vi "RecipeFile_Maker.vi"() -> ()   [LabVIEW 2014]
uses:
  <vilib>/Utility/file.llb/Write To Spreadsheet File (string).vi
panel:
  in  "RFSA_SettingFile_Path":path=path "C:/Gyuwon_Folder/SourceCodeFolder/1005_Gyu_RF_SourceProject_Msg/___SystemFiles/RFSA_Default_Setting.csv"
  in  "RFSG_SettingFile_Path":path=path "C:/Gyuwon_Folder/SourceCodeFolder/1005_Gyu_RF_SourceProject_Msg/___SystemFiles/RFSG_Default_Setting.csv"
  in  "RFSA_State":u16(ring) items=["RFSA_Init", "RFSA_Init_Servo", "Config_RFSA_AcqType_Vertical", "Config_RFSA_IQ_Acq", "Config_RFSA_Spectrum_Acq", "Config_RFSA_Trigger", "RFSA_Initiate", "RFSA_Fetch_IQ", "RFSA_Acq_Read_Spectrum", "RFSA_Acq_Read_IQ", "RFSA_Stop", "RFSA_Close", "Wait_Cmd", "Send_Cmd", "Exit"]
  in  "RFSG_State":u16(ring) items=["RFSG_Init", "RFSG_Init_Servo", "Config_ScriptWfm", "Config_Freq_Power_ExtGain", "Config_RFSG_Mode_CW", "Config_RFSG_Mode_Script", "RFSG_Write_Script", "RFSG_Initiate", "RFSG_Stop", "RFSG_Close", "Wait_Cmd", "Send_Cmd", "Exit"]
  in  "RFSA_Data":u16[](array[ring])=[0, 3, 1, 0, 0, 0] items=["None", "Config_RFSA_IQ_Acq", "Config_RFSA_Spectrum_Acq", "Config_RFSA_Vertical", "Config_RFSG"]
  in  "RFSA":u16[](array[ring])=[0, 2, 3, 5, 6, 7] items=["RFSA_Init", "RFSA_Init_Servo", "Config_RFSA_AcqType_Vertical", "Config_RFSA_IQ_Acq", "Config_RFSA_Spectrum_Acq", "Config_RFSA_Trigger", "RFSA_Initiate", "RFSA_Fetch_IQ", "RFSA_Acq_Read_Spectrum", "RFSA_Acq_Read_IQ", "RFSA_Stop", "RFSA_Close", "Wait_Cmd", "Send_Cmd", "Exit"]
  in  "RFSG_Data":u16[](array[ring])=[0, 4, 0, 0, 4, 0] items=["None", "Config_RFSA_IQ_Acq", "Config_RFSA_Spectrum_Acq", "Config_RFSA_Vertical", "Config_RFSG"]
  in  "RFSG":u16[](array[ring])=[0, 3, 2, 5, 6, 7] items=["RFSG_Init", "RFSG_Init_Servo", "Config_ScriptWfm", "Config_Freq_Power_ExtGain", "Config_RFSG_Mode_CW", "Config_RFSG_Mode_Script", "RFSG_Write_Script", "RFSG_Initiate", "RFSG_Stop", "RFSG_Close", "Wait_Cmd", "Send_Cmd", "Exit"]
  # "[ State 목록을 차후 변경될 때를 대비하여 enum으로 할 필요 있음 ]"
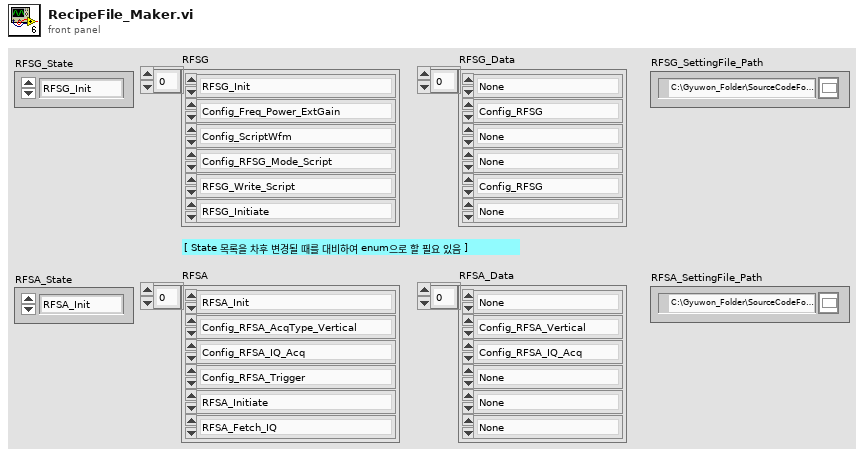
[diagram p1: front panel]
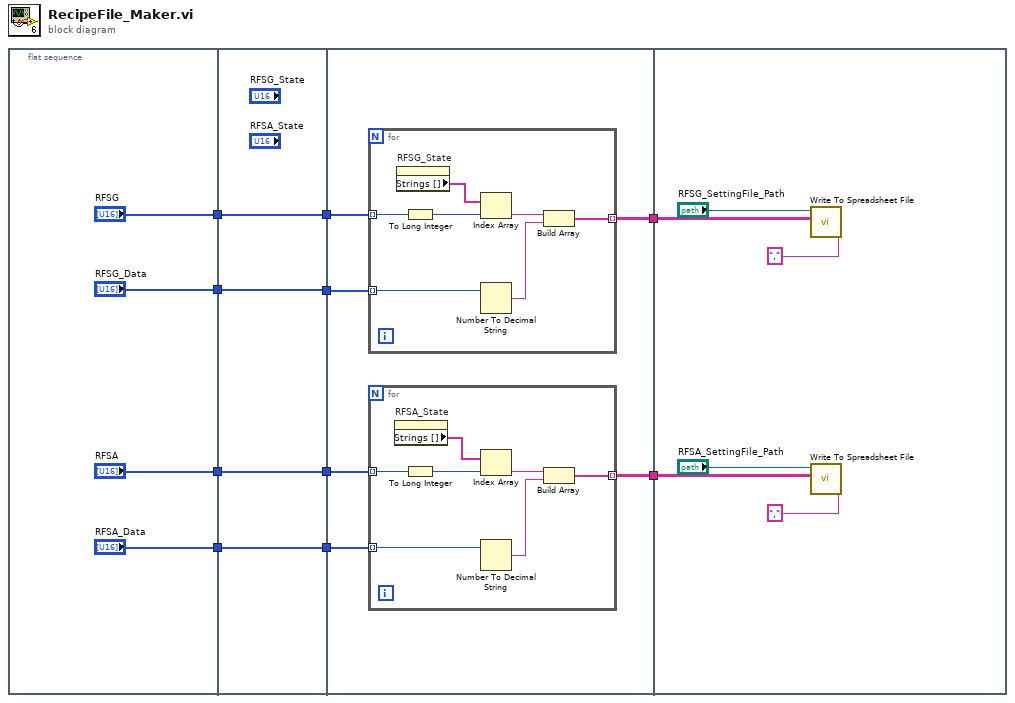
[diagram p0: block diagram]
diagram:
  n1 = flat-sequence {
    tunnel: ["RFSG"] -> w10
    tunnel: ["RFSG_Data"] -> w8
    tunnel: ["RFSA"] -> w5
    tunnel: ["RFSA_Data"] -> w1
    tunnel: w10 -> [w18]
    tunnel: [w18] -> w9
    tunnel: w8 -> [w17]
    tunnel: [w17] -> w7
    tunnel: w5 -> [w16]
    tunnel: [w16] -> w4
    tunnel: [w15] -> w2
    tunnel: w1 -> [w15]
    tunnel: w9 -> [w24]
    tunnel: w7 -> [w23]
    tunnel: [w22] -> w6
    tunnel: w4 -> [w21]
    tunnel: [w20] -> w3
    tunnel: w2 -> [w19]
    tunnel: w6 -> [w44]
    tunnel: w3 -> [w40]
    frame #0 {
    }
    frame #1 {
    }
    frame #2 {
      n2 = for {
        tunnel: w24 -> [w37] mode=indexing
        tunnel: w23 -> [w35] mode=indexing
        tunnel: [w32] -> w22 mode=indexing
        n3 = property on="RFSG_State" class="Ring (strict)"() -> ("Strings []"=w38:string[])  [unwired: 2 in, 2 out]
        n4 = To Long Integer(number=w37) -> (32bit integer=w36:i32)
        n5 = Index Array(array=w38, index=w36) -> (element=w34:string)
        n6 = Number To Decimal String(number=w35) -> (decimal integer string=w33:string)  [unwired: 1 in]
        n7 = Build Array(w34, w33) -> (w32:string[])
      }
      n8 = for {
        tunnel: w21 -> [w31] mode=indexing
        tunnel: w19 -> [w29] mode=indexing
        tunnel: [w26] -> w20 mode=indexing
        n9 = property on="RFSA_State" class="Ring (strict)"() -> ("Strings []"=w25:string[])  [unwired: 2 in, 2 out]
        n10 = To Long Integer(number=w31) -> (32bit integer=w30:i32)
        n11 = Index Array(array=w25, index=w30) -> (element=w28:string)
        n12 = Number To Decimal String(number=w29) -> (decimal integer string=w27:string)  [unwired: 1 in]
        n13 = Build Array(w28, w27) -> (w26:string[])
      }
    }
    frame #3 {
      n14 = call-poly <vilib>:"Write To Spreadsheet File.vi"("delimiter (\\t)"="," ("delimiter (\\t)"), "2D data"=w44, "file path (dialog if empty)"="RFSG_SettingFile_Path") -> ()  [unwired: 5 in, 1 out]
      n15 = call-poly <vilib>:"Write To Spreadsheet File.vi"("delimiter (\\t)"="," ("delimiter (\\t)"), "2D data"=w40, "file path (dialog if empty)"="RFSA_SettingFile_Path") -> ()  [unwired: 5 in, 1 out]
    }
  }
